vi "to string.vi"(8 "error in":errorcluster, 11 "user tag bus module configuration In":refnum<class "user tag bus module configuration.lvclass">) -> (0 "error out":errorcluster, 1 "data":string, 2 "version":string, 3 "user tag bus module configuration Out":refnum<class "user tag bus module configuration.lvclass">)   [LabVIEW 2013, in "user tag bus module configuration.lvclass"]
doc: "Provides an interface for saving a module configuration to a file or other serialized data source. It is recommended that all children of this class store data in two sets--data required for its own initialization, and any data required for parent initialization--and that each implementation uses the <b>Call Parent Method</b> primitive to serialize parent information."
uses:
  user tag bus module configuration.lvclass
  <vilib>/NI/Tag Bus Module Framework/module configuration/TBM module configuration.lvclass
  user tag bus module configuration.lvclass/user tag bus module configuration.ctl
  <vilib>/NI/Tag Bus Module Framework/root configuration/unwrap data.vi
  <vilib>/NI/Tag Bus Module Framework/root configuration/TBM configuration.lvclass
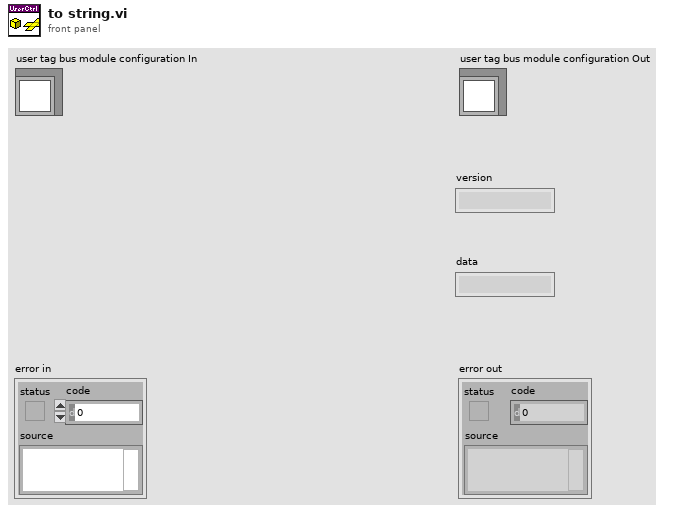
[diagram p1: front panel]
types:
  T1 = typedef "user tag bus module configuration.lvclass/state module configuration.ctl" = cluster{"fixed input":refnum<class "TBM channel.lvclass">, "fixed output":refnum<class "TBM channel.lvclass">, "initial state":u8}
  T2 = typedef "user tag bus module configuration.lvclass/control module configuration.ctl" = cluster{"name":string, "setpoint":refnum<class "TBM channel.lvclass">, "process variable":refnum<class "TBM channel.lvclass">, "output":refnum<class "TBM channel.lvclass">, "gains":T3, "output range":cluster{"output high":dbl, "output low":dbl}}
  T3 = typedef "user tag bus module configuration.lvclass/gains.ctl" = cluster{"Kp":dbl, "Ki":dbl, "Kd":dbl}
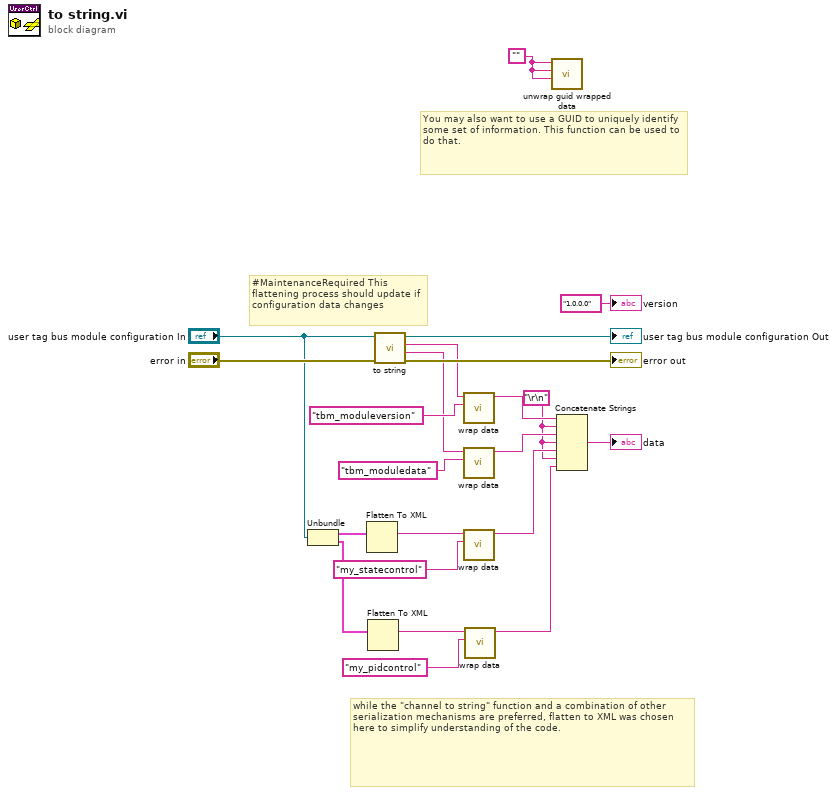
[diagram p0: block diagram]
diagram:
  w2 = "\r\n"
  w13 = ""
  # "while the \"channel to string\" function and a combination of other serialization mechanisms are preferred, flatten to XML was chosen here to simplify understanding of the code."
  # "You may also want to use a GUID to uniquely identify some set of information. This function can be used to do that."
  # "#MaintenanceRequired This flattening process should update if configuration data changes"
  n1 = Unbundle("user tag bus module configuration In") -> (w5:T1, w4:T2[])
  n2 = Flatten To XML(anything=w5) -> (xml string=w10:string)
  n3 = Flatten To XML(anything=w4) -> (xml string=w6:string)
  n4 = call-parent "to string.vi"("error in"="error in", "module configuration in"="user tag bus module configuration In") -> ("error out"=→"error out":errorcluster, "data"=w14:string, "version"=w15:string, "module configuration out"=→"user tag bus module configuration Out":refnum<class "user tag bus module configuration.lvclass">)  [unwired: 6 in]
  n5 = call <vilib>:"wrap data.vi"("identifier"="tbm_moduleversion" ("additional identifier"), "data to wrap"=w15) -> ("wrapped data"=w17:string)  [unwired: 9 in]
  n6 = call <vilib>:"wrap data.vi"("identifier"="tbm_moduledata" ("additional identifier"), "data to wrap"=w14) -> ("wrapped data"=w16:string)  [unwired: 9 in]
  n7 = call <vilib>:"wrap data.vi"("identifier"="my_statecontrol" ("additional identifier"), "data to wrap"=w10) -> ("wrapped data"=w9:string)  [unwired: 9 in]
  n8 = call <vilib>:"wrap data.vi"("identifier"="my_pidcontrol" ("additional identifier"), "data to wrap"=w6) -> ("wrapped data"=w3:string)  [unwired: 9 in]
  n9 = call <vilib>:"unwrap guid wrapped data.vi"("identifier"=w13, "uuid"=w13, "data to unwrap"=w13) -> ()  [unwired: 7 in, 2 out]
  n10 = Concatenate Strings(w17, w2, w16, w2, w9, w2, w3) -> (→"data":string)
  "version" <- "1.0.0.0" ("version")
